vi "Vector Drive.vi"(8 "error in":errorcluster, 10 "Drive Angle (radians)":dbl, 11 "Drive Magnitude":dbl) -> (0 "error out":errorcluster, 2 "Forward":dbl, 3 "Strafe":dbl)   [LabVIEW 2016]
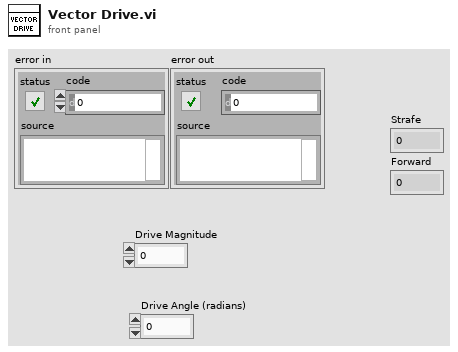
[diagram p1: front panel]
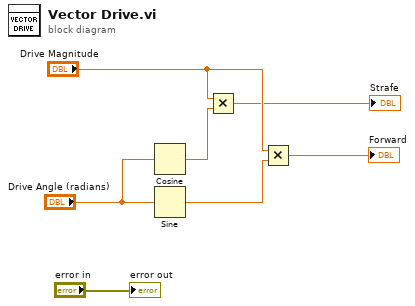
[diagram p0: block diagram]
diagram:
  n1 = Cosine(x="Drive Angle (radians)") -> (cos(x)=w4:dbl)
  n2 = Sine(x="Drive Angle (radians)") -> (sin(x)=w7:dbl)
  n3 = Multiply(x="Drive Magnitude", y=w4) -> (x*y=→"Strafe":dbl)
  n4 = Multiply(x="Drive Magnitude", y=w7) -> (x*y=→"Forward":dbl)
  "error out" <- "error in"
